vi "KI6221.vi"() -> ()   [LabVIEW 2025] (continued)
                                n1889 = Insert Into Array(array=w3447, index=1, new element=w3439) -> (w3446:string[])
                                n1890 = call "VisaVarReplace.vi"("Replace Array"=w3446, "Search Array"=string[] ["<DATASTART>", "<DATACOUNT>"], "GPIB Array"=w3451) -> ("GPIB Array OUT"=w3450:string[])
                                n1891 = case shown="True" w3437 {
                                tunnel: 1 ("index") -> [w3469 _]
                                tunnel: [w3468 ""] -> w3459
                                tunnel: [w3467 FALSE] -> w3458
                                tunnel: [w3465 errorcluster {"status"=FALSE, "code"=0, "source"=""} ("error out 15")] -> w3457
                                tunnel: w3456 -> [w3463 _]
                                tunnel: w3454 -> [w3462 _]
                                tunnel: w3450 -> [w3461 _]
                                frame False {
                                n1892 = call "VISAreadWrite.vi"("error in (no error)"=w3462, "GPIB INDEX Array"=i32[] [19], "GPIB ARRAY"=w3461, "VISA REFERENCE"=w3463) -> ("error out 15"=w3465:errorcluster, "Read Buffer Array"=w3466:string[])
                                n1893 = Index Array(array=w3466, index=w3469) -> (element=w3468:string)
                                n1894 = Unbundle(w3465) -> ("source"=w3464:string)  [unwired: 2 out]
                                n1895 = Match Pattern(string=w3464, regular expression="-1073807339") -> (offset past match=w3472:i32)  [unwired: 1 in, 3 out]
                                n1896 = Equal?(x=w3472, y=-1) -> (x = y?=w3467:bool)
                                }
                                frame True {
                                }
                                }
                                }
                                }
                                }
                                frame True {
                                }
                                }
                                }
                                }
                                frame Error {
                                n1897 = call "RUN DELTA ERROR6"() -> ("error out"=w3571:errorcluster)  [unwired: 10 in, 1 out]
                                n1898 = call "VISAreadWrite.vi"("error in (no error)"=w3571, "GPIB INDEX Array"=i32[] [18], "GPIB ARRAY"=w3569, "VISA REFERENCE"=w3568) -> ()  [unwired: 2 out]
                                }
                                }
                                n1899 = Array Subset(array=w3307, index (col)=4 ("index"), length (col)=1 ("length")) -> (w3306:string[][])  [unwired: 2 in]
                                n1900 = Fract/Exp String To Number(string=w3306) -> (number=w3335:dbl[][])  [unwired: 3 in, 1 out]
                                n1901 = Array Max & Min(array=w3335) -> (max value=w3281:dbl, min value=w3334:dbl)  [unwired: 2 out]
                                n1902 = Greater?(x=w3281, y=1e+30) -> (0:w3280:bool)
                                n1903 = call "Volt range problem"("Enable"=w3280) -> ()  [unwired: 9 in, 2 out]
                                n1904 = Equal?(x=w3334, y=w3281) -> (x = y?=w3333:bool)
                                n1905 = Equal To 0?(x=w3281) -> (x = 0?=w3332:bool)
                                n1906 = And(x=w3333, y=w3332) -> (x .and. y?=w3331:bool)
                                n1907 = call "Volt range problem"("Enable"=w3331) -> ()  [unwired: 9 in, 2 out]
                                }
                                frame True {
                                n1908 = Not(x=w3583) -> (.not. x?=w3584:bool)
                                n1909 = And(x=w3585, y=w3584) -> (x .and. y?=w3586:bool)
                                n1910 = call "No Nanovoltmeter present"("Enable"=w3586) -> ()  [unwired: 9 in, 2 out]
                                n1911 = call "No 6221 responding"("Enable"=w3583) -> ()  [unwired: 9 in, 2 out]
                                }
                                }
                                n1912 = property on="ABORT PULSE" class="Bool (strict)"() -> (error out=w3216:errorcluster, "Value"=w3219:bool)  [unwired: 2 in, 1 out]
                                n1913 = case shown="True" w3213 {
                                tunnel: w3218 -> [_ w3242]
                                tunnel: w3217 -> [_ w3241]
                                tunnel: w3216 -> [w3238 w3240]
                                tunnel: [w3238 w3239] -> w3215
                                frame False {
                                }
                                frame True {
                                n1914 = call "VISAreadWrite.vi"("error in (no error)"=w3240, "GPIB INDEX Array"=i32[] [21], "GPIB ARRAY"=w3241, "VISA REFERENCE"=w3242) -> ("error out 15"=w3239:errorcluster)  [unwired: 1 out]
                                }
                                }
                                n1915 = property on="Advanced Operation Tab" class="TabCtl (strict)"(error in=w3215, "Disabled"=0 ("Numeric 2")) -> (error out=→"DELTA SCPI ERROR 2":errorcluster)  [unwired: 1 in, 1 out]
                              }
                            }
                          }
                        }
                      }
                      frame True {
                        # "Update graph with demo data..."
                        n1916 = Add(x=u16 3, y=w3588) -> (x+y=w3592:u16)
                        n1917 = Index Array(array=w3590, index (col)=w3589) -> (element=w3594:string[])  [unwired: 1 in]
                        n1918 = Index Array(array=w3590, index (col)=w3592) -> (element=w3593:string[])  [unwired: 1 in]
                        n1919 = Array Size(array=w3593) -> (size(s)=w3591:i32)
                        n1920 = case shown="1, Default" w3591 {
                          tunnel: w3594 -> [_ w3604]
                          tunnel: w3593 -> [_ w3603]
                          tunnel: w3591 -> [_ w3602]
                          tunnel: w3590 -> [_ w3599]
                          tunnel: [FALSE w3598] -> w3587
                          frame 0 {
                          }
                          frame 1, Default {
                            w3601 = dbl[] []
                            n1921 = while {
                              tunnel: w3604 -> [w3630] mode=indexing
                              tunnel: w3603 -> [w3629] mode=indexing
                              shift-right: [w3622] -> _
                              shift-left: w3601 -> [w3627]
                              shift-right: [w3624] -> _
                              shift-left: w3601 -> [w3625]
                              tunnel: w3602 -> [w3618]
                              tunnel: w3599 -> [w3615]
                              shift-right: [w3605] -> _
                              shift-left: string[][] [] -> [w3616]
                              tunnel: [w3612] -> w3598
                              i -> [w3607]
                              stop <- w3613 stop-if-true
                              n1922 = Decrement(x=w3618) -> (x-1=w3620:i32)
                              n1923 = Fract/Exp String To Number(string=w3630) -> (number=w3628:dbl)  [unwired: 3 in, 1 out]
                              n1924 = Fract/Exp String To Number(string=w3629) -> (number=w3626:dbl)  [unwired: 3 in, 1 out]
                              n1925 = Index Array(array=w3615, index (row)=w3607) -> (element=w3614:string[])  [unwired: 1 in]
                              n1926 = Equal?(x=w3620, y=w3607) -> (x = y?=w3619:bool)
                              n1927 = Build Array (concatenate)(w3625, w3626) -> (w3624:dbl[])
                              n1928 = Build Array (concatenate)(w3627, w3628) -> (w3622:dbl[])
                              n1929 = Decrement(x=w3618) -> (x-1=w3617:i32)
                              n1930 = Equal?(x=w3617, y=w3607) -> ()  [unwired: 1 out]
                              n1931 = call "Convert to Dynamic Data3"("Array"=w3622) -> ("Dynamic Data Type"=w3621:dynamicdata)  [unwired: 3 in]
                              n1932 = call "Convert to Dynamic Data4"("Array"=w3624) -> ("Dynamic Data Type"=w3623:dynamicdata)  [unwired: 3 in]
                              n1933 = Divide(x=w3607, y=80) -> (x/y=w3609:dbl)
                              n1934 = Insert Into Array(array=w3616, index (row)=w3607, new element=w3614) -> (w3605:string[][])  [unwired: 1 in]
                              "PULSE DATA SHEET" <- w3605
                              n1935 = Round To Nearest(number=w3609) -> (nearest integer value=w3608:dbl)
                              n1936 = Equal?(x=w3609, y=w3608) -> (x = y?=w3610:bool)
                              n1937 = call "Build XY Graph3"("Y Input"=w3623, "X Input"=w3621) -> ("XY Graph"=w3611:cluster{"Y":dbl[], "Y":dbl[]}[])  [unwired: 8 in, 1 out]
                              n1938 = property on="ABORT PULSE" class="Bool (strict)"() -> ("Value"=w3612:bool)  [unwired: 2 in, 2 out]
                              n1939 = case shown="True" w3610 {
                                frame False {
                                }
                                frame True {
                                n1940 = Wait (ms)(milliseconds to wait=u16 1500 ("x")) -> ()  [unwired: 1 out]
                                }
                              }
                              n1941 = property on="Pulsed IV Graph" class="XYGraph (strict)"("Value"=w3611) -> ()  [unwired: 2 in, 2 out]
                              n1942 = Or(x=w3612, y=w3619) -> (x .or. y?=w3613:bool)
                            }
                          }
                        }
                      }
                    }
                    n1943 = case shown="True" w3133 {
                      frame False {
                      }
                      frame True {
                        n1944 = invoke on="PULSE DATA SHEET" class="Tbl" method="Reinit To Default"() -> ()  [unwired: 3 in, 3 out]
                        n1945 = invoke on="Pulsed IV Graph" class="XYGraph (strict)" method="Reinit To Default"() -> ()  [unwired: 3 in, 3 out]
                      }
                    }
                    n1946 = property on="ABORT PULSE" class="Bool (strict)"(error in=w3136, "Value"=FALSE, "Disabled"=2) -> (error out=w3132:errorcluster)  [unwired: 1 in, 1 out]
                    n1947 = property on="X Axis:" class="Ring (strict)"(error in=w3132, "Disabled"=w3111) -> (error out=w3131:errorcluster)  [unwired: 1 in, 1 out]
                    n1948 = property on="Y Axis:" class="Ring (strict)"(error in=w3131, "Disabled"=w3111) -> (error out=w3115:errorcluster)  [unwired: 1 in, 1 out]
                    n1949 = property on="RUN PULSE" class="Bool"(error in=w3115, "Disabled"=w3111) -> (error out=w3112:errorcluster)  [unwired: 1 in, 1 out]
                    n1950 = property on="Advanced Operation Tab" class="TabCtl (strict)"(error in=w3112, "Page Selector Visible"=w3101) -> (error out=w3102:errorcluster)  [unwired: 1 in, 1 out]
                    n1951 = property on="Main Tabs" class="TabCtl (strict)"(error in=w3102, "Page Selector Visible"=w3101) -> ()  [unwired: 1 in, 2 out]
                  }
                }
                n1952 = property on="X Axis:" class="Ring (strict)"() -> ("Value"=w3069:u16, "Strings []"=w3071:string[])  [unwired: 2 in, 2 out]
                n1953 = property on="Y Axis:" class="Ring (strict)"() -> ("Value"=w3068:u16, "Strings []"=w3070:string[])  [unwired: 2 in, 2 out]
                n1954 = local read "X AXIS LAST -PULSE"() -> (w3066:i32)
                n1955 = local read "Y AXIS LAST -PULSE"() -> (w3065:i32)
                n1956 = Equal?(x=w3065, y=w3068) -> (x = y?=w3072:bool)
                n1957 = Equal?(x=w3069, y=w3066) -> (x = y?=w3073:bool)
                n1958 = And(x=w3073, y=w3072) -> (x .and. y?=w3074:bool)
                n1959 = case shown="False" w3074 {
                  tunnel: w3069 -> [w3087 _]
                  tunnel: w3068 -> [w3086 _]
                  tunnel: w3071 -> [w3091 _]
                  tunnel: w3070 -> [w3090 _]
                  frame False {
                    n1960 = Add(x=w3086, y=3) -> (x+y=w3092:i32)
                    n1961 = property on="PULSE DATA SHEET" class="Tbl (strict)"() -> ("Value"=w3099:string[][])  [unwired: 2 in, 2 out]
                    n1962 = Index Array(array=w3099, index (col)=w3087) -> (element=w3098:string[])  [unwired: 1 in]
                    n1963 = Index Array(array=w3099, index (col)=w3092) -> (element=w3095:string[])  [unwired: 1 in]
                    n1964 = Index Array(array=w3091, index=w3087) -> (element=w3089:string)
                    n1965 = Fract/Exp String To Number(string=w3098) -> (number=w3097:dbl[])  [unwired: 3 in, 1 out]
                    n1966 = Fract/Exp String To Number(string=w3095) -> (number=w3094:dbl[])  [unwired: 3 in, 1 out]
                    n1967 = Index Array(array=w3090, index=w3086) -> (element=w3088:string)
                    n1968 = property on="Pulsed IV Graph" class="XYGraph (strict)"("X Scale.Name Label.Text"=w3089, "Y Scale.Name Label.Text"=w3088) -> ()  [unwired: 2 in, 2 out]
                    n1969 = call "Convert to Dynamic Data10"("Array"=w3097) -> ("Dynamic Data Type"=w3096:dynamicdata)  [unwired: 3 in]
                    n1970 = call "Convert to Dynamic Data9"("Array"=w3094) -> ("Dynamic Data Type"=w3093:dynamicdata)  [unwired: 3 in]
                    n1971 = call "Build XY Graph6"("Y Input"=w3093, "X Input"=w3096) -> ("XY Graph"=→"Pulsed IV Graph":cluster{"Y":dbl[], "Y":dbl[]}[])  [unwired: 8 in, 1 out]
                    "X AXIS LAST -PULSE" <- w3087
                    "Y AXIS LAST -PULSE" <- w3086
                  }
                  frame True {
                  }
                }
                n1972 = case shown="True" "CLEAR DATA PULSE" {
                  frame False {
                  }
                  frame True {
                    n1973 = invoke on="PULSE DATA SHEET" class="Table" method="Reinit To Default"() -> ()  [unwired: 3 in, 3 out]
                    n1974 = invoke on="Pulsed IV Graph" class="XYGraph (strict)" method="Reinit To Default"() -> ()  [unwired: 3 in, 3 out]
                  }
                }
                n1975 = local read "PULSE FILTER"() -> (w3064:u16)
                n1976 = case shown="0" w3064 {
                  tunnel: [FALSE TRUE] -> w3063
                  frame 0 {
                  }
                  frame 1, Default {
                  }
                }
                n1977 = property on="Pulse Filter Count" class="DigNum (strict)"("Visible"=w3063) -> ()  [unwired: 2 in, 2 out]
              }
              frame "Delta Mode Measurements", Default {
                # "Update graph when x-axis, y-axis \ncontrols are updated by the user."
                # "Referenced, but unconnected controls..."
                # "Enable num cycles with INF selection"
                # "save data function creates files..."
                # "Fliter visible..."
                # "Clear data button"
                n1978 = case shown="True" "RUN DELTA" {
                  frame False {
                  }
                  frame True {
                    w3758 = TRUE
                    w3756 = FALSE
                    w3785 = "%s" ("format string")
                    w3766 = 0 ("Numeric 2")
                    w3769 = u16 2 ("x")
                    # "SETUP GUI FOR DELTA MODE RUN"
                    n1979 = local read "Current Test File:"() -> (w3760:path)
                    n1980 = property on="ABORT DELTA" class="Bool (strict)"("Disabled"=u16 0 ("x"), "Value"=FALSE) -> (error out=w3794:errorcluster)  [unwired: 2 in, 1 out]
                    n1981 = property on="X Axis:" class="Ring (strict)"("Disabled"=w3769) -> ("Value"=w3795:u16, "Strings []"=w3796:string[])  [unwired: 2 in, 2 out]
                    n1982 = Index Array(array=w3796, index=w3795) -> (element=w3765:string)
                    n1983 = property on="Y Axis:" class="Ring (strict)"("Disabled"=w3769) -> ("Value"=w3797:u16, "Strings []"=w3798:string[])  [unwired: 2 in, 2 out]
                    n1984 = Index Array(array=w3798, index=w3797) -> (element=w3764:string)
                    n1985 = property on="Delta Mode Resistance Graph" class="XYGraph (strict)"("X Scale.Name Label.Text"=w3765, "Y Scale.Name Label.Text"=w3764) -> ()  [unwired: 2 in, 2 out]
                    n1986 = Equal?(x=w3760, y=path "") -> (x = y?=w3774:bool)
                    n1987 = case shown="True" w3774 {
                      tunnel: w3760 -> [w3806 _]
                      tunnel: [w3801 w3809] -> w3773
                      frame False {
                        n1988 = Path To String(path=w3806) -> (string=w3804:string)
                        n1989 = Search/Split String(string=w3804, search string/char (-)=".") -> (substring before match=w3803:string)  [unwired: 1 in, 2 out]
                        n1990 = Concatenate Strings(w3803, "_deltadata.kdf" ("search string/char (-)")) -> (w3800:string)
                        n1991 = String To Path(string=w3800) -> (path=w3801:path)
                      }
                      frame True {
                        n1992 = property on="Default path" class="Path"() -> ("Value"=w3807:path)  [unwired: 2 in, 2 out]
                        n1993 = Build Path(base path=w3807, name or relative path="DefaultTestFile_deltadata.cfg" ("file path (dialog if empty)")) -> (appended path=w3809:path)
                      }
                    }
                    n1994 = call <vilib>:"Read Lines From File.vi"("convert eol? (no:F)"=TRUE, "file path (dialog if empty)"=w3773, "number of lines (all:-1)"=-1) -> ("line string"=w3783:string)  [unwired: 3 in, 3 out]
                    n1995 = Match Pattern(string=w3783, regular expression="\n") -> (before substring=w3781:string, match substring=w3780:string, after substring=w3778:string)  [unwired: 1 in, 1 out]
                    n1996 = Concatenate Strings(w3781, w3780) -> (w3779:string)
                    n1997 = Spreadsheet String To Array(format string=w3785, spreadsheet string=w3779, array type (2D Dbl)=string[] []) -> ()  [unwired: 1 in, 1 out]
                    n1998 = Spreadsheet String To Array(format string=w3785, spreadsheet string=w3778, array type (2D Dbl)=string[][] []) -> (array=w3772:string[][])  [unwired: 1 in]
                    n1999 = property on="Main Tabs" class="TabCtl (strict)"("Page Selector Visible"=w3756) -> (error out=w3757:errorcluster)  [unwired: 2 in, 1 out]
                    n2000 = property on="Advanced Operation Tab" class="TabCtl (strict)"(error in=w3757, "Page Selector Visible"=w3756) -> (error out=w3768:errorcluster)  [unwired: 1 in, 1 out]
                    n2001 = property on="RUN DELTA" class="Bool"(error in=w3768, "Disabled"=w3769) -> (error out=w3762:errorcluster)  [unwired: 1 in, 1 out]
                    n2002 = invoke on="Delta Mode Resistance Graph" class="XYGraph (strict)" method="Reinit To Default"(error in=w3762) -> (error out=w3763:errorcluster)  [unwired: 2 in, 2 out]
                    n2003 = invoke on="Delta Mode Measurement Data" class="Table" method="Reinit To Default"(error in=w3763) -> (error out=w3770:errorcluster)  [unwired: 2 in, 2 out]
                    n2004 = property on="DEMO MODE" class="Bool (strict)"(error in=w3770) -> ("Value"=w3799:bool)  [unwired: 1 in, 2 out]
                    n2005 = case shown="False" w3799 {
                      tunnel: w3772 -> [_ w4133]
                      tunnel: w3795 -> [w3814 w4134]
                      tunnel: w3797 -> [w3813 w4139]
                      tunnel: w3794 -> [w3820 w4132]
                      tunnel: [w3820 w4132] -> w3792
                      tunnel: [w3819 w4131] -> w3789
                      frame False {
                        # "Checks for correct inputs...\nNO CONFLICTS GOES TO TRUE\nON NEXT CASE."
                        # "Make sure a NVMeter is selected."
                        # "REAL INSTRUMENT COMMUNICATION AFTER CONFLICT CHECKS"
                        n2006 = property on="High Current (Amps)" class="DigNum (strict)"() -> ("Value"=w3812:dbl)  [unwired: 2 in, 2 out]
                        n2007 = property on="Low Current (Amps)" class="DigNum (strict)"() -> ("Value"=w3811:dbl)  [unwired: 2 in, 2 out]
                        n2008 = property on="Select the nanovoltmeter model number:" class="Ring (strict)"() -> ("Value"=w3817:u16)  [unwired: 2 in, 2 out]
                        n2009 = Greater?(x=w3817, y=u16 1 ("x")) -> (0:w3815:bool)
                        n2010 = Not Equal?(x=w3812, y=w3811) -> (x != y?=w3810:bool)
                        n2011 = And(x=w3810, y=w3815) -> (x .and. y?=w3816:bool)
                        n2012 = case shown="False" w3816 {
                          tunnel: [FALSE w3832] -> w3819
                          tunnel: w3815 -> [w3822 _]
                          tunnel: w3814 -> [_ w3831]
                          tunnel: w3813 -> [_ w3830]
                          tunnel: w3810 -> [w3821 _]
                          frame False {
                            n2013 = case shown="False" w3822 {
                              frame False {
                                n2014 = One Button Dialog(message="To run a delta mode test, both a current source and\na nanovoltmeter must be connected and configured in\nthe instrument communication panel.") -> (true=w3824:bool)  [unwired: 1 in]
                                n2015 = case shown="False" w3824 {
                                frame False {
                                }
                                frame True, Default {
                                }
                                }
                              }
                              frame True {
                              }
                            }
                            n2016 = case shown="False" w3821 {
                              frame False {
                                n2017 = One Button Dialog(message="To run a test the High Current and Low Current values must be different. Change a value, then click RUN again.") -> (true=w3826:bool)  [unwired: 1 in]
                                n2018 = case shown="False" w3826 {
                                frame False {
                                }
                                frame True, Default {
                                n2019 = property on="High Current (Amps)" class="DigNum (strict)"("Key Focus"=TRUE) -> ()  [unwired: 2 in, 2 out]
                                }
                                }
                              }
                              frame True {
                              }
                            }
                          }
                          frame True {
                            (unwired) "Preparing instrument communication. Make certain device is correctly connected\nto the instruments, then click OK. "
                            # "ACTUAL DATA COMMUNICATION"
                            n2020 = case shown="True" "Case Constant\n(See Context Help) 7" {
                              tunnel: [FALSE w3840] -> w3832
                              tunnel: w3831 -> [_ w3843]
                              tunnel: w3830 -> [_ w3842]
                              frame False {
                              }
                              frame True {
                                # "TEST FOR MODEL PRESENT AT\nVISA RESOURCE..."
                                # "no NV"
                                # "NOT 6221"
                                n2021 = property on="6220 VISA" class="VISAName"() -> ("Value"=w3838:refnum<visa-resource-name>)  [unwired: 2 in, 2 out]
                                n2022 = property on="GPIB Array" class="Arr (strict)"() -> ("Value"=w3837:string[])  [unwired: 2 in, 2 out]
                                n2023 = call "VISAreadWrite.vi"("GPIB INDEX Array"=i32[] [0, 12], "GPIB ARRAY"=w3837, "VISA REFERENCE"=w3838) -> ("error out 15"=→"error out 16":errorcluster, "Read Buffer Array"=w3849:string[])  [unwired: 1 in]
                                n2024 = Index Array(array=w3849, index=1) -> (element=w3854:string)
                                n2025 = Match Pattern(string=w3854, regular expression="MODEL 622") -> (offset past match=w3846:i32)  [unwired: 1 in, 3 out]
                                n2026 = Equal?(x=w3846, y=-1) -> (x = y?=w3844:bool)
                                n2027 = Index Array(array=w3849, index=3) -> (element=w3848:string)
                                n2028 = Decimal String To Number(string=w3848) -> (number=w3847:i32)  [unwired: 2 in, 1 out]
                                n2029 = Equal To 0?(x=w3847) -> (x = 0?=w3845:bool)
                                n2030 = Or(x=w3845, y=w3844) -> (x .or. y?=w3835:bool)
                                n2031 = case shown="False" w3835 {
                                tunnel: w3845 -> [_ w4128]
                                tunnel: w3844 -> [_ w4126]
                                tunnel: w3837 -> [w3939 _]
                                tunnel: w3838 -> [w3885 _]
                                tunnel: w3843 -> [w3901 _]
                                tunnel: w3842 -> [w3900 _]
                                tunnel: [TRUE FALSE] -> w3834
                                frame False {
                                w3902 = string[][] []
                                # "TEST FOR DATA IN BUFFER. GET DATA AND PLACE ON GRAPH AND DATASHEET. REPEAT UNTIL ALL DATA \nHAS BEEN RETRIEVED. (WAIT 2 sec. between checking the buffer."
                                # "SEND SCPI SETUP STRINGS"
                                # "CREATE SCPI STRINGS FROM CONTROL VARIABLES"
                                n2032 = property on="High Current (Amps)" class="DigNum (strict)"() -> ("Value"=w3868:dbl)  [unwired: 2 in, 2 out]
                                n2033 = property on="Current Source \nVoltage Compliance (V)" class="DigNum (strict)"() -> ("Value"=w3934:dbl)  [unwired: 2 in, 2 out]
                                n2034 = property on="Number of cycles" class="DigNum (strict)"() -> ("Value"=w3875:i32)  [unwired: 2 in, 2 out]
                                n2035 = property on="INFINITE DELTA CYCLES" class="Bool (strict)"() -> ("Value"=w3930:bool)  [unwired: 2 in, 2 out]
                                n2036 = property on="FILTER" class="Ring (strict)"() -> ("Value"=w3932:u16)  [unwired: 2 in, 2 out]
                                n2037 = property on="Low Current (Amps)" class="DigNum (strict)"() -> ("Value"=w3867:dbl)  [unwired: 2 in, 2 out]
                                n2038 = property on="Filter\nCount" class="DigNum (strict)"() -> ("Value"=w3886:i32)  [unwired: 2 in, 2 out]
                                n2039 = property on="Voltage Measure Range" class="Ring (strict)"() -> ("Value"=w3933:dbl)  [unwired: 2 in, 2 out]
                                n2040 = Negate(x=w3867) -> (-x=w3888:dbl)
                                n2041 = property on="Delay (mS) - settle time" class="DigNum (strict)"() -> ("Value"=w3937:dbl)  [unwired: 2 in, 2 out]
                                n2042 = Number To Exponential String(number=w3933) -> (E-format string=w3915:string)  [unwired: 3 in]
                                n2043 = property on="DAMPING" class="Bool (strict)"() -> ("Value"=w3911:bool)  [unwired: 2 in, 2 out]
                                n2044 = property on="Measurement Integration (NPLCs)" class="DigNum (strict)"() -> ("Value"=w3935:dbl)  [unwired: 2 in, 2 out]
                                n2045 = Subtract(x=w3868, y=w3867) -> (x-y=w3889:dbl)
                                n2046 = Absolute Value(x=w3868) -> (abs(x)=w3866:dbl)
                                n2047 = Absolute Value(x=w3867) -> (abs(x)=w3865:dbl)
                                n2048 = Number To Exponential String(number=w3868) -> (E-format string=w3919:string)  [unwired: 3 in]
                                n2049 = Equal?(x=w3888, y=w3868) -> (x = y?=w3887:bool)
                                n2050 = Number To Exponential String(number=w3867) -> (E-format string=w3918:string)  [unwired: 3 in]
                                n2051 = Number To Exponential String(number=w3934) -> (E-format string=w3914:string)  [unwired: 3 in]
                                n2052 = Divide(x=w3937, y=1000.0) -> (x/y=w3938:dbl)
                                n2053 = Boolean To (0,1)(Boolean=w3911) -> (0, 1=w3910:i16)
                                n2054 = Number To Exponential String(number=w3935) -> (E-format string=w3913:string)  [unwired: 3 in]
                                n2055 = Number To Exponential String(number=w3938) -> (E-format string=w3912:string)  [unwired: 3 in]
                                n2056 = Number To Decimal String(number=w3886) -> (decimal integer string=w3931:string)  [unwired: 1 in]
                                n2057 = Divide(x=w3889, y=2.0) -> (x/y=w3881:dbl)
                                n2058 = Number To Decimal String(number=w3910) -> (decimal integer string=w3909:string)  [unwired: 1 in]
                                n2059 = case shown="False" w3930 {
                                tunnel: [w4114 "INF"] -> w3917
                                tunnel: w3875 -> [w4113 _]
                                frame False {
                                n2060 = Number To Decimal String(number=w4113) -> (decimal integer string=w4114:string)  [unwired: 1 in]
                                }
                                frame True {
                                (unwired) 0 ("Value")
                                }
                                }
                                n2061 = case shown="0, Default" w3932 {
                                tunnel: w3931 -> [w4117 w4121 w4124]
                                tunnel: [w4117 w4121 w4124] -> w3908
                                tunnel: ["MOV" "MOV" "REP"] -> w3916
                                tunnel: ["0" "1" "1"] -> w3904
                                frame 0, Default {
                                }
                                frame 1 {
                                }
                                frame 2 {
                                }
                                }
                                n2062 = Greater?(x=w3866, y=w3865) -> (0:w3870:bool)
                                n2063 = Select(t=w3866, s=w3870, f=w3865) -> (s? t:f=w3869:dbl)
                                n2064 = Number To Exponential String(number=w3869) -> (E-format string=w3871:string)  [unwired: 3 in]
                                n2065 = Insert Into Array(array=string[] [] ("Replace Array"), new element=w3919) -> (w3928:string[])  [unwired: 1 in]
                                n2066 = Insert Into Array(array=w3928, new element=w3918) -> (w3927:string[])  [unwired: 1 in]
                                n2067 = Insert Into Array(array=w3927, new element=w3917) -> (w3926:string[])  [unwired: 1 in]
                                n2068 = Insert Into Array(array=w3926, new element=w3916) -> (w3925:string[])  [unwired: 1 in]
                                n2069 = Insert Into Array(array=w3925, new element=w3915) -> (w3924:string[])  [unwired: 1 in]
                                n2070 = Insert Into Array(array=w3924, new element=w3914) -> (w3906:string[])  [unwired: 1 in]
                                n2071 = Insert Into Array(array=w3906, new element=w3871) -> (w3923:string[])  [unwired: 1 in]
                                n2072 = Insert Into Array(array=w3923, new element=w3913) -> (w3922:string[])  [unwired: 1 in]
                                n2073 = Insert Into Array(array=w3922, new element=w3912) -> (w3921:string[])  [unwired: 1 in]
                                n2074 = Insert Into Array(array=w3921, new element=w3909) -> (w3920:string[])  [unwired: 1 in]
                                n2075 = Insert Into Array(array=w3920, new element=w3908) -> (w3905:string[])  [unwired: 1 in]
                                n2076 = Insert Into Array(array=w3905, new element=w3904) -> (w3878:string[])  [unwired: 1 in]
                                n2077 = Add(x=u16 2, y=w3900) -> (x+y=w3899:u16)
                                n2078 = local read "Setup String"() -> (w3879:string)
                                n2079 = Insert Into Array(array=w3878, new element=w3879) -> (w3877:string[])  [unwired: 1 in]
                                n2080 = call "VisaVarReplace.vi"("Replace Array"=w3877, "Search Array"=string[] ["<DELTAHIGH>", "<DELTALOW>", "<DELTANUMCYCLE>", "<DELTAFILTERTYPE>", "<DELTAVOLTRANGE>", "<DELTACOMP>", "<DELTACURRRANGE>", "<DELTANPLC>", "<DELTADELAY>", "<DELTADAMPING>", "<DELTAFILTERCOUNT>", "<DELTAFILTERSTATE>", "<SETUPSTRING>"], "GPIB Array"=w3939) -> ("GPIB Array OUT"=w3884:string[])
                                n2081 = call "VISAreadWrite.vi"("GPIB INDEX Array"=i32[] [16], "GPIB ARRAY"=w3884, "VISA REFERENCE"=w3885) -> ("error out 15"=w3883:errorcluster)  [unwired: 1 in, 1 out]
                                n2082 = case shown="No Error" w3883 {
                                tunnel: w3885 -> [w3951 w4109]
                                tunnel: w3884 -> [w3950 w4110]
                                tunnel: w3875 -> [w3949 _]
                                tunnel: w3902 -> [_ _]
                                tunnel: dbl[] [] -> [w3948 _]
                                tunnel: w3902 -> [w3947 _]
                                tunnel: w3901 -> [w3946 _]
                                tunnel: w3899 -> [w3945 _]
                                tunnel: [w3942 string[][] [["", "", "", "1"], ["", "", "", ""], ["", "", "", ""], ["", "", "", "1"]]] -> w3897
                                tunnel: w3881 -> [w3944 _]
                                tunnel: w3887 -> [w3943 _]
                                tunnel: 0.0 -> [w3941 _]
                                frame No Error {
                                n2083 = while {
                                tunnel: w3951 -> [w3965]
                                tunnel: w3950 -> [w3964]
                                tunnel: w3949 -> [w3963]
                                tunnel: w3948 -> [w3961]
                                tunnel: w3946 -> [w3959]
                                tunnel: w3945 -> [w3958]
                                tunnel: w3944 -> [w3957]
                                tunnel: w3943 -> [w3956]
                                shift-right: [w3954] -> w3942
                                shift-left: w3947 -> [w3960]
                                shift-right: [w3953] -> _
                                shift-left: w3941 -> [w3952]
                                stop <- w3962 stop-if-true
                                n2084 = case shown="False" "ABORT DELTA" {
                                tunnel: w3965 -> [w3982 _]
                                tunnel: w3964 -> [w3981 _]
                                tunnel: w3963 -> [w3979 _]
                                tunnel: [w3978 w4106] -> w3962
                                tunnel: w3961 -> [w3977 _]
                                tunnel: w3960 -> [w3976 _]
                                tunnel: [w3975 string[][] [["", "", "", "1"], ["", "", "", ""], ["", "", "", ""], ["", "", "", "1"]]] -> w3954
                                tunnel: w3959 -> [w3974 _]
                                tunnel: w3958 -> [w3973 _]
                                tunnel: w3957 -> [w3970 _]
                                tunnel: w3956 -> [w3969 _]
                                tunnel: "ABORT DELTA" -> [w3968 w4106]
                                tunnel: [w3967 w4104] -> w3953
                                tunnel: w3952 -> [w3966 w4104]
                                frame False {
                                n2085 = case shown="True" w3971 {
                                tunnel: w3980 -> [_ w4063]
                                tunnel: w3979 -> [_ w4060]
                                tunnel: [FALSE w4059] -> w3978
                                tunnel: w3977 -> [_ w4057]
                                tunnel: w3976 -> [_ w4035]
                                tunnel: [string[][] [["", "", "", ""], ["", "", "", ""], ["", "", "", ""], ["", "", "", "1"]] w4053] -> w3975
                                tunnel: w3974 -> [_ w4052]
                                tunnel: w3973 -> [_ w4051]
                                tunnel: w3972 -> [_ w4044]
                                tunnel: w3970 -> [_ w4043]
                                tunnel: w3969 -> [_ w4042]
                                tunnel: w3968 -> [_ w4041]
                                tunnel: [w4029 w4033] -> w3967
                                tunnel: w3966 -> [w4029 _]
                                frame False {
                                }
                                frame True {
                                n2086 = Decrement(x=w4060) -> (x-1=w4040:i32)
                                n2087 = Bundle(0, 0) -> (w4039:cluster{i32, i32})  [unwired: 1 in]
                                n2088 = Spreadsheet String To Array(delimiter (Tab)=",", format string="%e", spreadsheet string=w4044, array type (2D Dbl)=w4057) -> (array=w4056:dbl[])
                                n2089 = while {
                                tunnel: w4056 -> [w4077]
                                tunnel: [w4076] -> w4034
                                tunnel: w4043 -> [w4072]
                                tunnel: w4042 -> [w4073]
                                shift-right: [w4070] -> w4036
                                shift-left: string[][] [] -> [w4064]
                                i -> [w4069]
                                stop <- w4092 stop-if-true
                                w4085 = "," ("delimiter (Tab)")
                                n2090 = Array Size(array=w4064) -> (size(s)=w4067:i32[])
                                n2091 = Index Array(array=w4067, index=0) -> (element=w4065:i32)
                                n2092 = Multiply(x=4, y=w4065) -> (x*y=w4095:i32)
                                n2093 = Index Array(array=w4077, index=w4095) -> (element=w4071:dbl)
                                n2094 = Divide(x=w4071, y=w4072) -> (x/y=w4075:dbl)
                                n2095 = Increment(x=w4095) -> (x+1=w4093:i32)
                                n2096 = Index Array(array=w4077, index=w4093) -> (element=w4078:dbl)
                                n2097 = case shown="False" w4073 {
                                tunnel: ["" w4101] -> w4079
                                tunnel: w4072 -> [_ w4099]
                                tunnel: w4071 -> [_ w4098]
                                frame False {
                                }
                                frame True {
                                n2098 = Multiply(x=w4099, y=w4098) -> (x*y=w4100:dbl)
                                n2099 = Number To Engineering String(4:w4100) -> (0:w4101:string)  [unwired: 3 in]
                                }
                                }
                                n2100 = Increment(x=w4093) -> (x+1=w4094:i32)
                                n2101 = Reciprocal(x=w4075) -> (1/x=w4074:dbl)
                                n2102 = Index Array(array=w4077, index=w4094) -> ()  [unwired: 1 out]
                                n2103 = Increment(x=w4094) -> (x+1=w4090:i32)
                                n2104 = Array Size(array=w4077) -> (size(s)=w4068:i32)
                                n2105 = Index Array(array=w4077, index=w4090) -> (element=w4076:dbl)
                                n2106 = Increment(x=w4090) -> (x+1=w4091:i32)
                                n2107 = Number To Engineering String(4:w4078) -> (0:w4083:string)  [unwired: 3 in]
                                n2108 = Number To Engineering String(4:w4071) -> (0:w4081:string)  [unwired: 3 in]
                                n2109 = Number To Engineering String(4:w4074) -> (0:w4080:string)  [unwired: 3 in]
                                n2110 = Number To Engineering String(4:w4075) -> (0:w4082:string)  [unwired: 3 in]
                                n2111 = Greater Or Equal?(x=w4091, y=w4068) -> (x >= y?=w4092:bool)
                                n2112 = Number To Decimal String(number=w4076) -> (decimal integer string=w4084:string)  [unwired: 1 in]
                                n2113 = Concatenate Strings(w4084, w4085, w4083, w4085, w4082, w4085, w4081, w4085, w4080, w4085, w4079) -> (w4086:string)
                                n2114 = Spreadsheet String To Array(delimiter (Tab)=w4085, format string="%s", spreadsheet string=w4086, array type (2D Dbl)=string[] []) -> (array=w4087:string[])
                                n2115 = Insert Into Array(array=w4064, index (row)=w4069, new element=w4087) -> (w4070:string[][])  [unwired: 1 in]
                                }
                                n2116 = Insert Into Array(array=w4035, new element=w4036) -> (w4053:string[][])  [unwired: 2 in]
                                n2117 = Equal?(x=w4040, y=w4034) -> (x = y?=w4058:bool)
                                n2118 = Index Array(array=w4053, index (col)=w4052) -> (element=w4050:string[])  [unwired: 1 in]
                                n2119 = Fract/Exp String To Number(string=w4050) -> (number=w4048:dbl[])  [unwired: 3 in, 1 out]
                                n2120 = call "Convert to Dynamic Data5"("Array"=w4048) -> ("Dynamic Data Type"=w4047:dynamicdata)  [unwired: 3 in]
                                n2121 = property on="Delta Mode Measurement Data" class="Tbl (strict)"("Value"=w4053, "Edit Position"=w4039) -> ()  [unwired: 2 in, 2 out]
                                n2122 = Index Array(array=w4053, index (col)=w4051) -> (element=w4049:string[])  [unwired: 1 in]
                                n2123 = Fract/Exp String To Number(string=w4049) -> (number=w4046:dbl[])  [unwired: 3 in, 1 out]
                                n2124 = call "Convert to Dynamic Data11"("Array"=w4046) -> ("Dynamic Data Type"=w4045:dynamicdata)  [unwired: 3 in]
                                n2125 = call "Build XY Graph"("Y Input"=w4045, "X Input"=w4047) -> ("XY Graph"=w4061:cluster{"Y":dbl[], "Y":dbl[]}[])  [unwired: 8 in, 1 out]
                                n2126 = property on="Delta Mode Resistance Graph" class="XYGraph (strict)"("Value"=w4061) -> ()  [unwired: 2 in, 2 out]
                                n2127 = case shown="Error" w4063 {
                                tunnel: [w4102 TRUE] -> w4062
                                tunnel: w4041 -> [w4102 _]
                                frame No Error {
                                }
                                frame Error {
                                n2128 = call "RUN DELTA ERROR2"() -> ()  [unwired: 10 in, 2 out]
                                }
                                }
                                n2129 = Or(x=w4062, y=w4058) -> (x .or. y?=w4059:bool)
                                n2130 = Increment(x=w4034) -> (x+1=w4033:dbl)
                                }
                                }
                                n2131 = flat-sequence {
                                tunnel: w3981 -> [w3986]
                                tunnel: w3982 -> [w3987]
                                tunnel: [w3987] -> w3984
                                tunnel: [w3986] -> w3983
                                tunnel: [w4009] -> w3980
                                tunnel: [w4011] -> w3972
                                tunnel: [w4010] -> w3971
                                tunnel: w3984 -> [w4008]
                                tunnel: w3983 -> [w4003]
                                tunnel: w3966 -> [w3992]
                                frame #0 {
                                n2132 = Wait (ms)(milliseconds to wait=u32 2000) -> ()  [unwired: 1 out]
                                }
                                frame #1 {
                                n2133 = call "VISAreadWrite.vi"("GPIB INDEX Array"=i32[] [4], "GPIB ARRAY"=w4003, "VISA REFERENCE"=w4008) -> ("error out 15"=w4006:errorcluster, "Read Buffer Array"=w4004:string[])  [unwired: 1 in]
                                n2134 = Index Array(array=w4004, index=1) -> (element=w3994:string)
                                n2135 = Number To Decimal String(number=w3992) -> (decimal integer string=w3995:string)  [unwired: 1 in]
                                n2136 = Insert Into Array(array=string[] [] ("Replace Array"), index=0, new element=w3995) -> (w3999:string[])
                                n2137 = Decimal String To Number(string=w3994) -> (number=w3993:i32)  [unwired: 2 in, 1 out]
                                n2138 = Subtract(x=w3993, y=w3992) -> (x-y=w3989:dbl)
                                n2139 = Round To Nearest(number=w3989) -> (nearest integer value=w3988:dbl)
                                n2140 = Less Or Equal To 0?(x=w3988) -> (x <= 0?=w3990:bool)
                                n2141 = Number To Decimal String(number=w3988) -> (decimal integer string=w3991:string)  [unwired: 1 in]
                                n2142 = Insert Into Array(array=w3999, index=1, new element=w3991) -> (w3998:string[])
                                n2143 = call "VisaVarReplace.vi"("Replace Array"=w3998, "Search Array"=string[] ["<DATASTART>", "<DATACOUNT>"], "GPIB Array"=w4003) -> ("GPIB Array OUT"=w4002:string[])
                                n2144 = case shown="False" w3990 {
                                tunnel: 1 ("index") -> [w4021 _]
                                tunnel: [w4020 ""] -> w4011
                                tunnel: [w4019 FALSE] -> w4010
                                tunnel: [w4017 errorcluster {"status"=FALSE, "code"=0, "source"=""} ("error out 15")] -> w4009
                                tunnel: w4008 -> [w4015 _]
                                tunnel: w4006 -> [w4014 _]
                                tunnel: w4002 -> [w4013 _]
                                frame False {
                                n2145 = call "VISAreadWrite.vi"("error in (no error)"=w4014, "GPIB INDEX Array"=i32[] [19], "GPIB ARRAY"=w4013, "VISA REFERENCE"=w4015) -> ("error out 15"=w4017:errorcluster, "Read Buffer Array"=w4018:string[])
                                n2146 = Index Array(array=w4018, index=w4021) -> (element=w4020:string)
                                n2147 = Unbundle(w4017) -> ("source"=w4016:string)  [unwired: 2 out]
                                n2148 = Match Pattern(string=w4016, regular expression="-1073807339") -> (offset past match=w4024:i32)  [unwired: 1 in, 3 out]
                                n2149 = Equal?(x=w4024, y=-1) -> (x = y?=w4019:bool)
                                }
                                frame True {
                                }
                                }
                                }
                                }
                                }
                                frame True {
                                }
                                }
                                }
                                }
                                frame Error {
                                n2150 = call "RUN DELTA ERROR"() -> ("error out"=w4112:errorcluster)  [unwired: 10 in, 1 out]
                                n2151 = call "VISAreadWrite.vi"("error in (no error)"=w4112, "GPIB INDEX Array"=i32[] [18], "GPIB ARRAY"=w4110, "VISA REFERENCE"=w4109) -> ("error out 15"=→"error out 27":errorcluster)  [unwired: 1 out]
                                }
                                }
                                n2152 = Array Subset(array=w3897, index (col)=3 ("index"), length (col)=1 ("length")) -> (w3895:string[][])  [unwired: 2 in]
                                n2153 = Fract/Exp String To Number(string=w3895) -> (number=w3894:dbl[][])  [unwired: 3 in, 1 out]
                                n2154 = Array Max & Min(array=w3894) -> (max value=w3874:dbl, min value=w3893:dbl)  [unwired: 2 out]
                                n2155 = Equal?(x=w3893, y=w3874) -> (x = y?=w3892:bool)
                                n2156 = Equal To 0?(x=w3874) -> (x = 0?=w3891:bool)
                                n2157 = Greater?(x=w3874, y=1e+30) -> (0:w3872:bool)
                                n2158 = call "Volt range problem"("Enable"=w3872) -> ()  [unwired: 9 in, 2 out]
                                n2159 = And(x=w3892, y=w3891) -> (x .and. y?=w3890:bool)
                                n2160 = call "Volt range problem"("Enable"=w3890) -> ()  [unwired: 9 in, 2 out]
                                }
                                frame True {
                                n2161 = Not(x=w4126) -> (.not. x?=w4127:bool)
                                n2162 = And(x=w4128, y=w4127) -> (x .and. y?=w4129:bool)
                                n2163 = call "No Nanovoltmeter present"("Enable"=w4129) -> ()  [unwired: 9 in, 2 out]
                                n2164 = call "No 6220/6221 responding"("Enable"=w4126) -> ()  [unwired: 9 in, 2 out]
                                }
                                }
                                n2165 = property on="ABORT DELTA" class="Bool (strict)"() -> (error out=w3836:errorcluster, "Value"=w3840:bool)  [unwired: 2 in, 1 out]
                                n2166 = case shown="True" w3834 {
                                tunnel: [w3858 w3862] -> w3839
                                tunnel: w3838 -> [_ w3861]
                                tunnel: w3837 -> [_ w3860]
                                tunnel: w3836 -> [w3858 w3859]
                                frame False {
                                }
                                frame True {
                                n2167 = call "VISAreadWrite.vi"("error in (no error)"=w3859, "GPIB INDEX Array"=i32[] [17], "GPIB ARRAY"=w3860, "VISA REFERENCE"=w3861) -> ("error out 15"=w3862:errorcluster)  [unwired: 1 out]
                                }
                                }
                                n2168 = property on="Advanced Operation Tab" class="TabCtl (strict)"(error in=w3839, "Disabled"=0 ("Numeric 2")) -> (error out=→"DELTA SCPI ERROR":errorcluster)  [unwired: 1 in, 1 out]
                              }
                            }
                          }
                        }
                      }
                      frame True {
                        # "DEMO MODE PULL DATA AND REGRAPH/LOAD SHEET"
                        n2169 = Add(x=u16 2, y=w4139) -> (x+y=w4135:u16)
                        n2170 = Index Array(array=w4133, index (col)=w4134) -> (element=w4137:string[])  [unwired: 1 in]
                        n2171 = Index Array(array=w4133, index (col)=w4135) -> (element=w4136:string[])  [unwired: 1 in]
                        n2172 = Array Size(array=w4136) -> (size(s)=w4130:i32)
                        n2173 = case shown="1, Default" w4130 {
                          tunnel: w4137 -> [_ w4147]
                          tunnel: w4136 -> [_ w4146]
                          tunnel: w4130 -> [_ w4145]
                          tunnel: w4133 -> [_ w4142]
                          tunnel: [FALSE w4141] -> w4131
                          frame 0 {
                          }
                          frame 1, Default {
                            w4144 = dbl[] []
                            n2174 = while {
                              tunnel: w4147 -> [w4173] mode=indexing
                              tunnel: w4146 -> [w4172] mode=indexing
                              shift-right: [w4165] -> _
                              shift-left: w4144 -> [w4170]
                              shift-right: [w4167] -> _
                              shift-left: w4144 -> [w4168]
                              tunnel: w4145 -> [w4161]
                              tunnel: w4142 -> [w4158]
                              shift-right: [w4148] -> _
                              shift-left: string[][] [] -> [w4159]
                              tunnel: [w4155] -> w4141
                              i -> [w4149]
                              stop <- w4156 stop-if-true
                              n2175 = Decrement(x=w4161) -> (x-1=w4163:i32)
                              n2176 = Fract/Exp String To Number(string=w4173) -> (number=w4171:dbl)  [unwired: 3 in, 1 out]
                              n2177 = Fract/Exp String To Number(string=w4172) -> (number=w4169:dbl)  [unwired: 3 in, 1 out]
                              n2178 = Index Array(array=w4158, index (row)=w4149) -> (element=w4157:string[])  [unwired: 1 in]
                              n2179 = Equal?(x=w4163, y=w4149) -> (x = y?=w4162:bool)
                              n2180 = Divide(x=w4149, y=80) -> (x/y=w4152:dbl)
                              n2181 = Build Array (concatenate)(w4168, w4169) -> (w4167:dbl[])
                              n2182 = Round To Nearest(number=w4152) -> (nearest integer value=w4151:dbl)
                              n2183 = Build Array (concatenate)(w4170, w4171) -> (w4165:dbl[])
                              n2184 = Decrement(x=w4161) -> (x-1=w4160:i32)
                              n2185 = Equal?(x=w4152, y=w4151) -> (x = y?=w4153:bool)
                              n2186 = Equal?(x=w4160, y=w4149) -> ()  [unwired: 1 out]
                              n2187 = call "Convert to Dynamic Data2"("Array"=w4165) -> ("Dynamic Data Type"=w4164:dynamicdata)  [unwired: 3 in]
                              n2188 = call "Convert to Dynamic Data"("Array"=w4167) -> ("Dynamic Data Type"=w4166:dynamicdata)  [unwired: 3 in]
                              n2189 = case shown="True" w4153 {
                                frame False {
                                }
                                frame True {
                                n2190 = Wait (ms)(milliseconds to wait=u16 2000 ("x")) -> ()  [unwired: 1 out]
                                }
                              }
                              n2191 = Insert Into Array(array=w4159, index (row)=w4149, new element=w4157) -> (w4148:string[][])  [unwired: 1 in]
                              "Delta Mode Measurement Data" <- w4148
                              n2192 = call "Build XY Graph2"("Y Input"=w4166, "X Input"=w4164) -> ("XY Graph"=w4154:cluster{"Y":dbl[], "Y":dbl[]}[])  [unwired: 8 in, 1 out]
                              n2193 = property on="Delta Mode Resistance Graph" class="XYGraph (strict)"("Value"=w4154) -> ()  [unwired: 2 in, 2 out]
                              n2194 = property on="ABORT DELTA" class="Bool (strict)"() -> ("Value"=w4155:bool)  [unwired: 2 in, 2 out]
                              n2195 = Or(x=w4155, y=w4162) -> (x .or. y?=w4156:bool)
                            }
                          }
                        }
                      }
                    }
                    n2196 = case shown="True" w3789 {
                      frame False {
                      }
                      frame True {
                        n2197 = invoke on="Delta Mode Resistance Graph" class="XYGraph (strict)" method="Reinit To Default"() -> ()  [unwired: 3 in, 3 out]
                        n2198 = invoke on="Delta Mode Measurement Data" class="Tbl" method="Reinit To Default"() -> ()  [unwired: 3 in, 3 out]
                      }
                    }
                    n2199 = property on="ABORT DELTA" class="Bool (strict)"(error in=w3792, "Disabled"=2 ("Numeric 2"), "Value"=FALSE) -> (error out=w3787:errorcluster)  [unwired: 1 in, 1 out]
                    n2200 = property on="X Axis:" class="Ring (strict)"(error in=w3787, "Disabled"=w3766) -> (error out=w3786:errorcluster)  [unwired: 1 in, 1 out]
                    n2201 = property on="Y Axis:" class="Ring (strict)"(error in=w3786, "Disabled"=w3766) -> (error out=w3771:errorcluster)  [unwired: 1 in, 1 out]
                    n2202 = property on="RUN DELTA" class="Bool"(error in=w3771, "Disabled"=w3766) -> (error out=w3767:errorcluster)  [unwired: 1 in, 1 out]
                    n2203 = property on="Advanced Operation Tab" class="TabCtl (strict)"(error in=w3767, "Page Selector Visible"=w3758) -> (error out=w3759:errorcluster)  [unwired: 1 in, 1 out]
                    n2204 = property on="Main Tabs" class="TabCtl (strict)"(error in=w3759, "Page Selector Visible"=w3758) -> ()  [unwired: 1 in, 2 out]
                  }
                }
                n2205 = case shown="True" "DELTA DEMO" {
                  frame False {
                  }
                  frame True {
                    # "FILTER CAN NOT BE ABOVE 100. ADD'L ERROR CHECK"
                    n2206 = local read "Low Current (Amps)"() -> (w3670:dbl)
                    n2207 = local read "High Current (Amps)"() -> (w3671:dbl)
                    n2208 = local read "Filter\nCount"() -> (w3677:i32)
                    n2209 = local read "FILTER"() -> (w3675:u16)
                    n2210 = Greater?(x="Select the nanovoltmeter model number:", y=u16 1 ("x")) -> (0:w3678:bool)
                    n2211 = Greater?(x=101, y=w3677) -> (0:w3673:bool)
                    n2212 = Not Equal?(x=w3670, y=w3671) -> (x != y?=w3679:bool)
                    n2213 = Equal To 0?(x=w3675) -> (x = 0?=w3674:bool)
                    n2214 = Or(x=w3673, y=w3674) -> (x .or. y?=w3672:bool)
                    n2215 = Compound Arithmetic op=AND(w3679, w3678, w3672) -> (w3681:bool)
                    n2216 = case shown="False" w3681 {
                      tunnel: w3670 -> [_ w3702]
                      tunnel: w3671 -> [_ w3701]
                      tunnel: w3679 -> [w3685 _]
                      tunnel: w3678 -> [w3684 _]
                      tunnel: w3677 -> [_ w3700]
                      tunnel: w3672 -> [w3683 _]
                      tunnel: w3675 -> [_ w3699]
                      tunnel: w3671 -> [_ w3698]
                      tunnel: w3670 -> [_ w3697]
                      frame False {
                        n2217 = case shown="False" w3684 {
                          frame False {
                            n2218 = One Button Dialog(message="To run a delta mode test, both a current source and\na nanovoltmeter must be connected and configured in\nthe instrument communication panel.") -> (true=w3689:bool)  [unwired: 1 in]
                            n2219 = case shown="False" w3689 {
                              frame False {
                              }
                              frame True, Default {
                              }
                            }
                          }
                          frame True {
                          }
                        }
                        n2220 = case shown="False" w3685 {
                          frame False {
                            n2221 = One Button Dialog(message="To run a test the High Current and Low Current values must be different. Change a value, then click RUN again.") -> (true=w3691:bool)  [unwired: 1 in]
                            n2222 = case shown="False" w3691 {
                              frame False {
                              }
                              frame True, Default {
                                n2223 = property on="High Current (Amps)" class="DigNum (strict)"("Key Focus"=TRUE) -> ()  [unwired: 2 in, 2 out]
                              }
                            }
                          }
                          frame True {
                          }
                        }
                        n2224 = case shown="False" w3683 {
                          frame False {
                            n2225 = One Button Dialog(message="To run the delta mode demo the filter count must be 100 or fewer points.") -> (true=w3686:bool)  [unwired: 1 in]
                            n2226 = case shown="False" w3686 {
                              frame False {
                              }
                              frame True, Default {
                                n2227 = property on="Filter\nCount" class="DigNum (strict)"("Key Focus"=TRUE) -> ()  [unwired: 2 in, 2 out]
                              }
                            }
                          }
                          frame True {
                          }
                        }
                      }
                      frame True {
                        # "need to do tests for bad inputs.\nneed to generate these vars same\nas below.....\nneed to test no INSTR and others\ninside subvi."
                        n2228 = local read "Current Source \nVoltage Compliance (V)"() -> (w3722:dbl)
                        n2229 = local read "Measurement Integration (NPLCs)"() -> (w3716:dbl)
                        n2230 = local read "Delay (mS) - settle time"() -> (w3696:dbl)
                        n2231 = local read "6220 VISA"() -> (w3730:refnum<visa-resource-name>)
                        n2232 = local read "Setup String"() -> (w3724:string)
                        n2233 = Divide(x=w3696, y=1000.0) -> (x/y=w3694:dbl)
                        n2234 = local read "GPIB Array"() -> (w3729:string[])
                        n2235 = Number To Engineering String(4:w3716) -> (0:w3715:string)  [unwired: 3 in]
